vi "T7 Byte to Volts KAG_Old_AvgSlope.vi"(8 "error in":errorcluster, 10 "file (use dialog)":path=path "/Macintosh HD/Users/kgompertz/Desktop/JUM Data Log/untitled", 11 "Byte Data":u16[][](array[numeric])) -> (0 "error out":errorcluster, 3 "Float Data":dbl[][](array[numeric]))   [LabVIEW 2022 SP3]
doc: "Apply T7 calibration contents (read from flash memory chip) to convert U16 data to raw voltage data.\n\nThere is a plot on the right hidden by the front panel edge."
uses:
  T7 Stream Globals KAG.vi
  <vilib>/Utility/file.llb/Write Delimited Spreadsheet (DBL).vi
panel:
  out "Waveform Graph":dbl[][](graph)
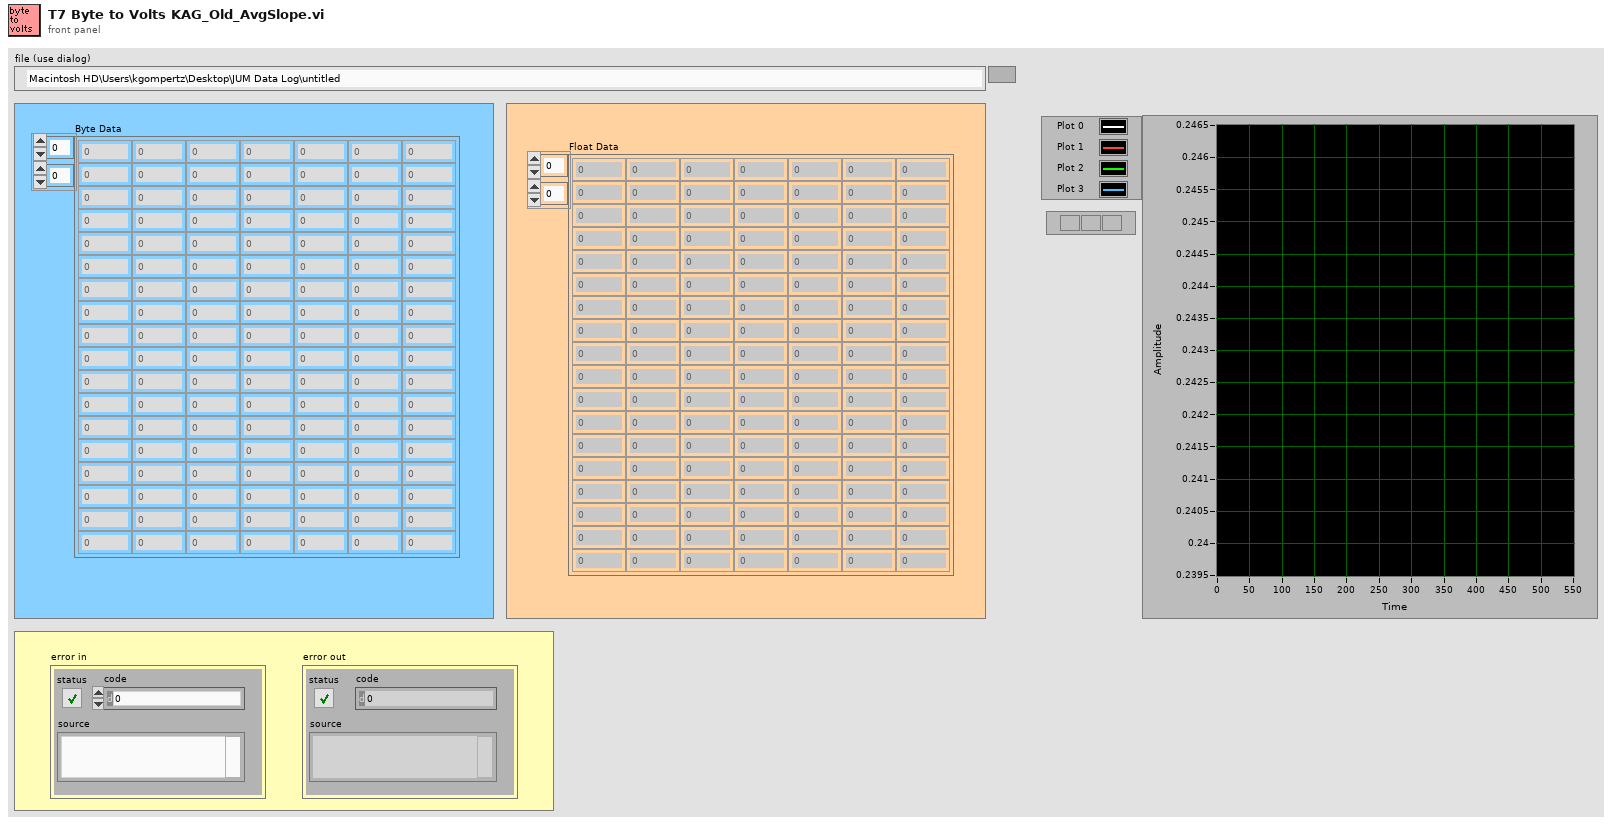
[diagram p1: front panel]
types:
  T1 = cluster{"Channel":u32, "BipGain":u32, "Input Config":string}[]
  T2 = cluster{"PSlope":dbl, "NSlope":dbl, "AvgSlope":dbl, "Center":dbl, "Offset":dbl}[]
  T3 = cluster{"PSlope":dbl, "NSlope":dbl, "AvgSlope":dbl, "Center":dbl, "Offset":dbl}
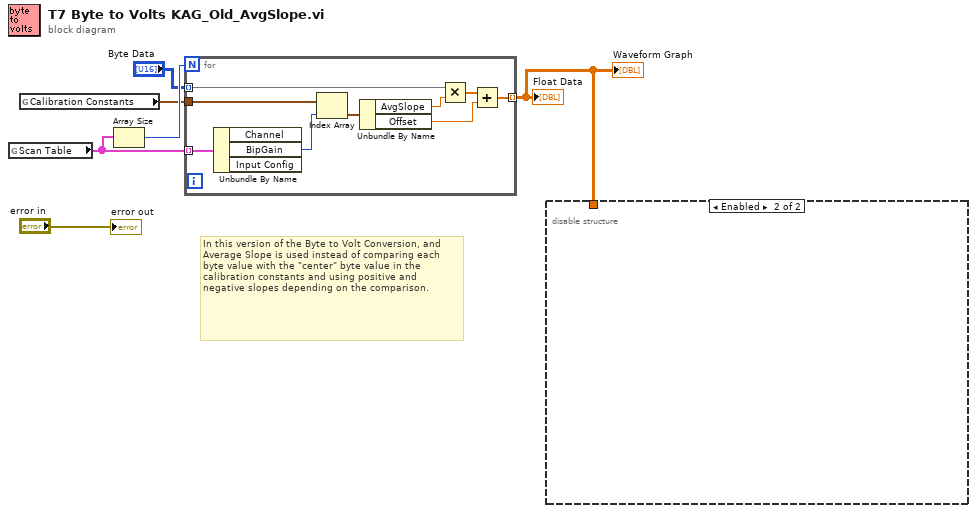
[diagram p0: block diagram]
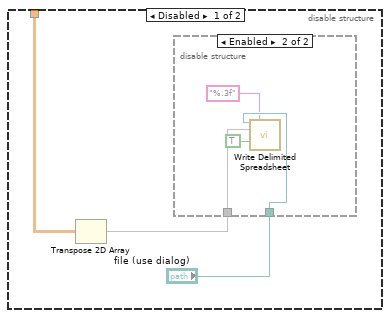
[diagram p2: hidden frame]
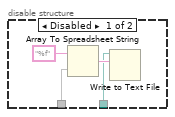
[diagram p3: hidden frame]
diagram:
  # "In this version of the Byte to Volt Conversion, and Average Slope is used instead of comparing each byte value with the \"center\" byte value in the calibration constants and using positive and negative slopes depending on the comparison."
  n1 = global read "T7 Stream Globals KAG.vi" "Scan Table"() -> (w6:T1)
  n2 = global read "T7 Stream Globals KAG.vi" "Calibration Constants"() -> (w4:T2)
  n3 = Array Size(array=w6) -> (size(s)=w5:i32)
  n4 = for {
    N: w5 -> [_]
    tunnel: w6 -> [w15] mode=indexing
    tunnel: w4 -> [w14]
    tunnel: "Byte Data" -> [w11] mode=indexing
    tunnel: [w8] -> w1 mode=indexing
    n5 = Unbundle By Name(w15) -> ("BipGain"=w7:u32)  [unwired: 2 out]
    n6 = Index Array(array=w14, index=w7) -> (element=w13:T3)
    n7 = Unbundle By Name(w13) -> ("AvgSlope"=w12:dbl, "Offset"=w10:dbl)
    n8 = Multiply(x=w11, y=w12) -> (x*y=w9:dbl[])
    n9 = Add(x=w9, y=w10) -> (x+y=w8:dbl[])
  }
  "Float Data" <- w1
  "Waveform Graph" <- w1
  n10 = disable-structure shown="Enabled" {
    disable-tunnel: w1 -> [w18 _]
    frame Disabled {
      n11 = Transpose 2D Array(2D array=w18) -> (transposed array=w17:dbl[][])
      n12 = disable-structure shown="Enabled" {
        disable-tunnel: w17 -> [w22 w26]
        disable-tunnel: "file (use dialog)" -> [w20 w24]
        frame Disabled {
          n13 = Array To Spreadsheet String(array=w22, 3:"%f" ("format string")) -> (spreadsheet string=w21:string)  [unwired: 1 in]
          n14 = Write to Text File(file (use dialog)=w20, text=w21) -> ()  [unwired: 2 in, 3 out]
        }
        frame Enabled {
          n15 = call-poly <vilib>:"Write Delimited Spreadsheet.vi"("file path (dialog if empty)"=w24, "format (%.3f)"="%.3f", "2D data"=w26, "append to file? (new file:F)"=TRUE ("append to file? (F)")) -> ()  [unwired: 10 in, 2 out]
        }
      }
    }
    frame Enabled {
    }
  }
  "error out" <- "error in"
